vi "Open menu object parameters.vi"(8 "error in (no error)":errorcluster, 10 "Object name":string, 11 "Mag Lab Measure Interface in":refnum<class "Mag Lab Measure UI.lvclass">) -> (0 "error out":errorcluster, 3 "Mag Lab Measure Interface out":refnum<class "Mag Lab Measure UI.lvclass">)   [LabVIEW 2015, in "Mag Lab Measure UI.lvclass"]
uses:
  Mag Lab Measure UI.lvclass
  <vilib>/ActorFramework/Actor/Actor.lvclass/Actor.ctl
  Mag Lab Measure Base Messages/Open sub-object parameters Msg/Open nested object parameters Msg.lvclass/Open nested object parameters Msg.ctl
  <vilib>/ActorFramework/Message Enqueuer/Message Enqueuer.lvclass/Message Enqueuer.ctl
  <vilib>/ActorFramework/Message Enqueuer/Enqueue.vi
  <vilib>/ActorFramework/Message Priority Queue/Priority Enqueue.vi
  Mag Lab Measure Base Messages/Open sub-object parameters Msg/Open nested object parameters Msg.lvclass
  <vilib>/ActorFramework/Actor/Actor.lvclass
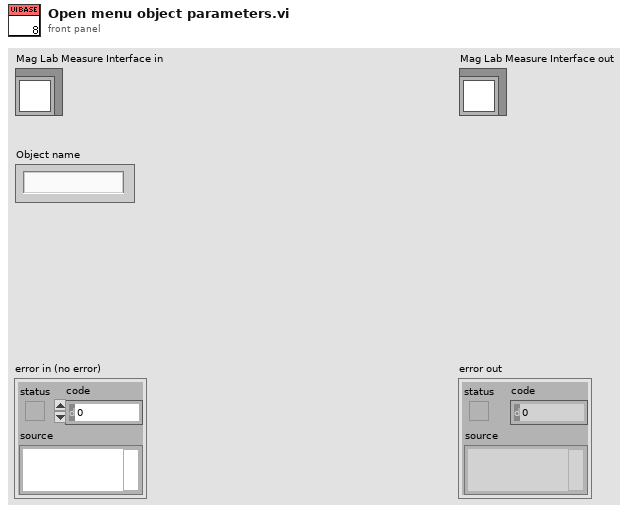
[diagram p1: front panel]
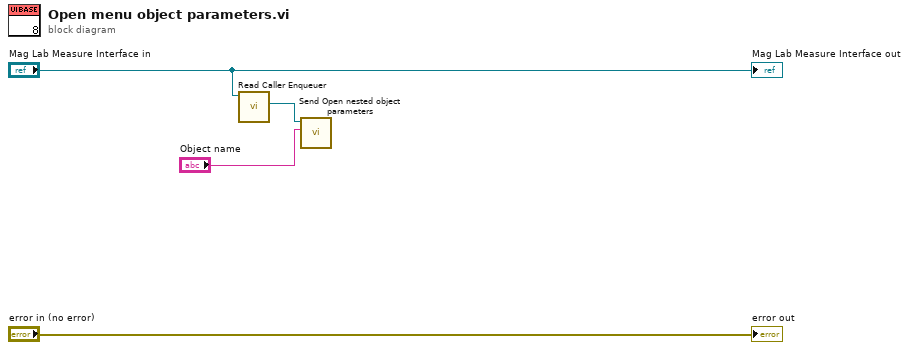
[diagram p0: block diagram]
diagram:
  n1 = call <vilib>:"Read Caller Enqueuer.vi"("Actor"="Mag Lab Measure Interface in") -> ("Caller Enqueuer"=w2:refnum<class "Message Enqueuer.lvclass">)  [unwired: 10 in]
  n2 = call "Send Open nested object parameters.vi"("Object name"="Object name", "Message Enqueuer"=w2) -> ()  [unwired: 8 in, 2 out]
  "error out" <- "error in (no error)"
  "Mag Lab Measure Interface out" <- "Mag Lab Measure Interface in"
